vi "Reset Encoders.vi"(7 "Description":string, 8 "Command Info In":T1) -> (0 "Command Info Out":T1)   [LabVIEW 2017]
doc: "This VI notifies the subsystem to the new setpoint."
uses:
  <vilib>/Rock Robotics/WPI/Framework/Command Status Info.ctl
  <vilib>/Rock Robotics/WPI/Framework/Completion Status.ctl
  <vilib>/Rock Robotics/WPI/Framework/Completion Notifier.ctl
  Implementation/Drive Setpoints.ctl
  Implementation/Drive Operations.ctl
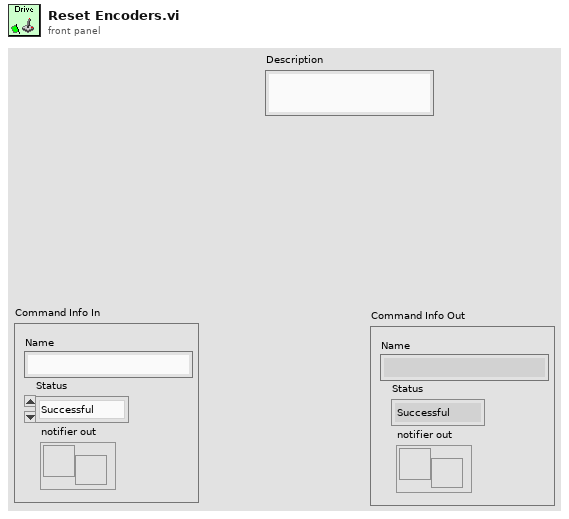
[diagram p1: front panel]
types:
  T1 = typedef "Command Status Info.ctl" = cluster{"Name":string, "Status":T2, "notifier out":T3}
  T2 = typedef "Completion Status.ctl" = enum16{"Successful", "Aborted", "Incomplete"}
  T3 = typedef "Completion Notifier.ctl" = refnum<notifier>
  T4 = typedef "Drive Setpoints.ctl" = cluster{"Operation":T5, "X Setpoint":dbl, "Y Setpoint":dbl, "Duration":dbl, "Z Setpoint":dbl, "Tracks":bool, "Gyro":dbl, "POV":i16, "Distance(feet)":dbl, "AutoTrack Toggle":bool, "Collsision Detection":bool, "Reset Encoder":bool, "MP File Name":string}
  T5 = typedef "Drive Operations.ctl" = enum16{"Reserve", "Read Current", "Reset Motors VBus", "Motion Profile run", "Immediate Robot Centric", "Drive for Time Robot Centric", "Immediate Field Centric", "Drive For Time Field Centric", "Button Adjust", "Set Motors Motion Profile", "Reset Encoders", "Motion Profile Enable", "Drive for Distance"}
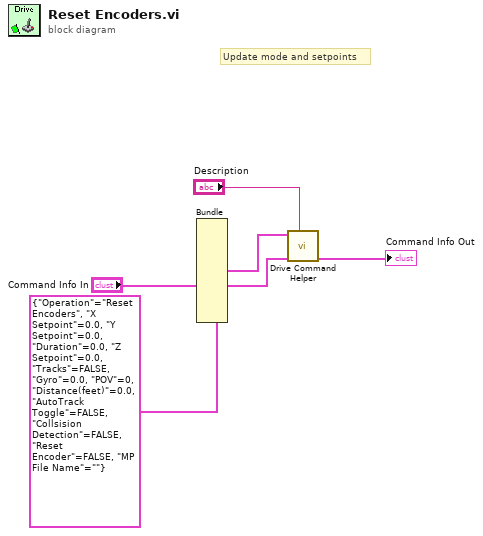
[diagram p0: block diagram]
diagram:
  # "Update mode and setpoints"
  n1 = Bundle(cluster=T4 {"Operation"=enum."Reset Encoders", "X Setpoint"=0.0, "Y Setpoint"=0.0, "Duration"=0.0, "Z Setpoint"=0.0, "Tracks"=FALSE, "Gyro"=0.0, "POV"=0, "Distance(feet)"=0.0, "AutoTrack Toggle"=FALSE, "Collsision Detection"=FALSE, "Reset Encoder"=FALSE, "MP File Name"=""} ("SubSystem Data")) -> (w1:T4)  [unwired: 13 in]
  n2 = call "Drive Command Helper.vi"("Description"="Description", "Command Info In"="Command Info In", "SubSystem Data"=w1) -> ("Command Info Out"=→"Command Info Out":T1)  [unwired: 7 in, 1 out]
